vi "WinHostToFlexRIO.vi"() -> ()   [LabVIEW 2013]
uses:
  <vilib>/userdefined/High Color/nirio_resource_hc.ctl
  <vilib>/FPGAPlugInAG/PXIe-7966R/niLvFpga_Open_PXIe-7966R.vi
  <vilib>/FPGAPlugInAG/PXIe-7966R/niLvFpga_Reset_PXIe-7966R.vi
  <vilib>/FPGAPlugInAG/PXIe-7966R/niLvFpga_Run_PXIe-7966R.vi
  <vilib>/Utility/error.llb/Error Cluster From Error Code.vi
  <vilib>/rvi/errors/niLvFpgaAdjustHostInterfaceError.vi
  <vilib>/rvi/interface/common/niFpgaWaitOnOcc.vi
  <vilib>/FPGAPlugInAG/PXIe-7966R/niLvFpga_Close_PXIe-7966R.vi
  <vilib>/rvi/interface/nirviOpenFPGA/nirviOpenFPGA.xnode
  FPGA Bitfiles/PXIe-7966R-FlexRIOMod5761_v1_1.lvbitx
  FlexRIO5761.vi
  <vilib>/rvi/interface/nirviMethod/nirviMethod.xnode
  <vilib>/rvi/interface/nirviReadWriteControl/nirviReadWriteControl.xnode
  Control 1.ctl
  <vilib>/rvi/interface/nirviCloseFPGA/nirviCloseFPGA.xnode
  <vilib>/rvi/errors/niLvFpgaMergeErrorWithErrorCode.vi
  NiFpgaLv.dll
  <vilib>/FPGAPlugInAG/PXIe-7966R/niLvFpga_ReadFifo_PXIe-7966R.vi
  <vilib>/Analysis/NI_AALPro.lvlib
  <vilib>/FPGAPlugInAG/PXIe-7966R/niLvFpga_ConfigureFifo_PXIe-7966R.vi
  <vilib>/FPGAPlugInAG/PXIe-7966R/niLvFpga_StartFifo_PXIe-7966R.vi
panel:
  in  "SGSignalType1":enum16{"DC", "Sine", "Square", "Triangle"}(ring)
  out "Power spectrum graph":dynamicdata(graph)
  in  "SGAmp1":u16
  in  "AO1":i32
  in  "SGPhase1":u32
  in  "SGFreq1":u32
  in  "SGUpdateRate1":u32
  in  "AOEnable1":bool
  in  "FlexRIO device":T1
  out "DMA0 output":dynamicdata(graph)
  in  "SGSignalType0":enum16{"DC", "Sine", "Square", "Triangle"}(ring)
  in  "stop":bool
  out "auxAI9":i16
  out "SGNo":u8
  in  "SGAmp0":u16
  in  "SamplingRate0":u32=10000
  in  "DMATtoHOSTEnable0":bool
  in  "AO0":i16
  in  "SGFreq0":u32
  in  "SGPhase0":u32
  in  "SGUpdateRate0":u32=10000000
  in  "AOEnable0":bool
  in  "DebugMode":bool
  in  "DAQStartStop":bool
  out "error out":errorcluster
  out "DMATtoHOSTBlockNWords":u16[](array[numeric])
  out "DMATtoHOSTSampleSize":u8[](array[numeric])
  out "DMATtoHOSTNCh":u16[](array[numeric])
  out "DMATtoHOSTFrameType":u8[](array[numeric])
  out "DevProfile":u8
  out "DevTemp":i16
  out "DevQualityStatus":u8
  out "Fref":u32
  out "RIOAdapterCorrect":bool
  out "Expected IO Module ID":u32
  out "InsertedIOModule ID":u32
  out "FPGAVIversion":u8[](array[numeric])
  out "Platform":enum8{"FlexRIO", "cRIO", "RSeries"}(ring)
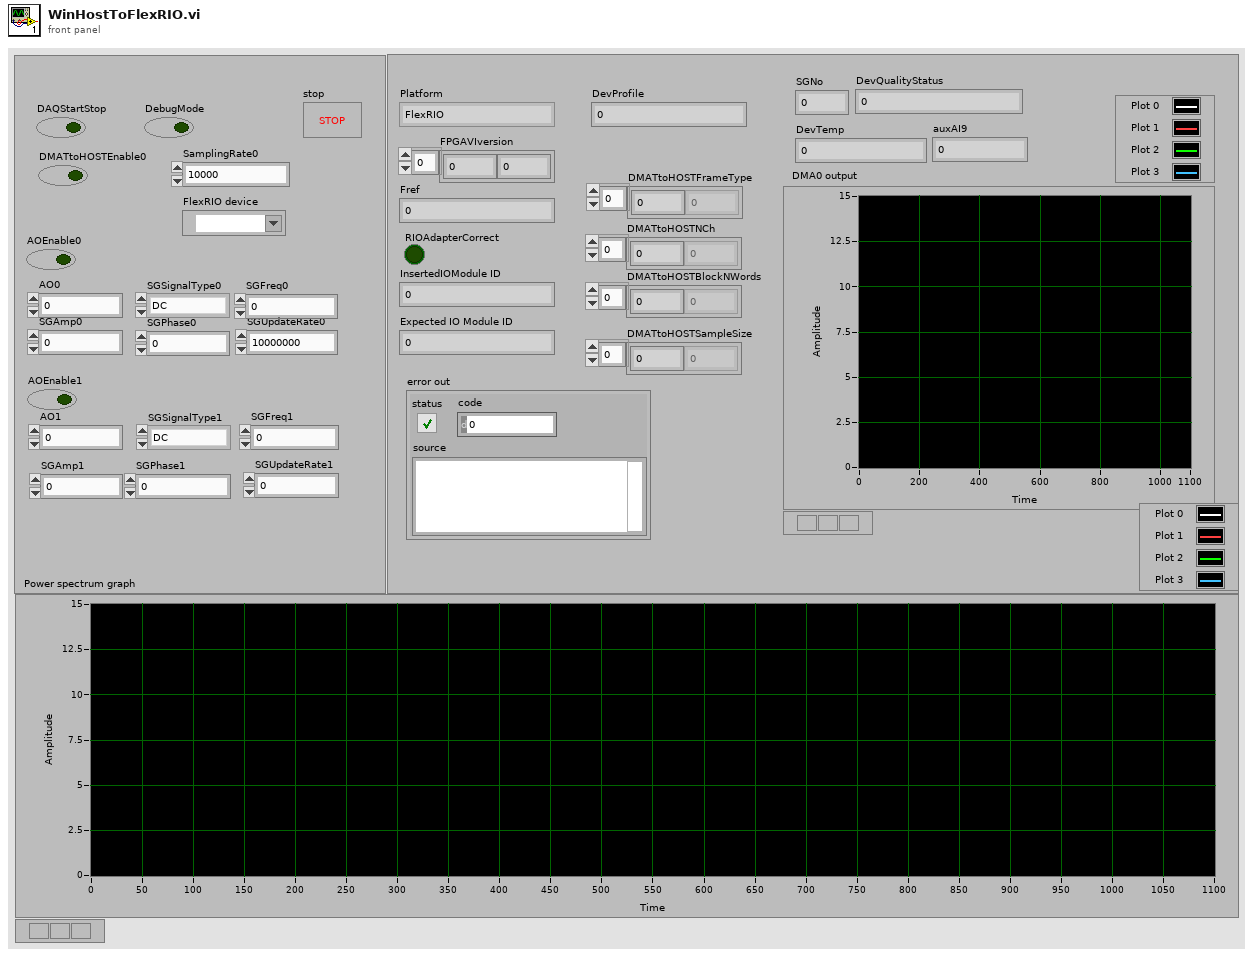
[diagram p1: front panel]
types:
  T1 = typedef "nirio_resource_hc.ctl" = tag
  T2 = enum16{"DAQ-CPU", "IMAQ-CPU", "DAQ-GPU", "IMAQ-GPU"}
  T3 = typedef "Control 1.ctl" = u16
  T4 = cluster{"Timeout":u8, "Timeout":T3, "Timeout":u8, "Timeout":u16}
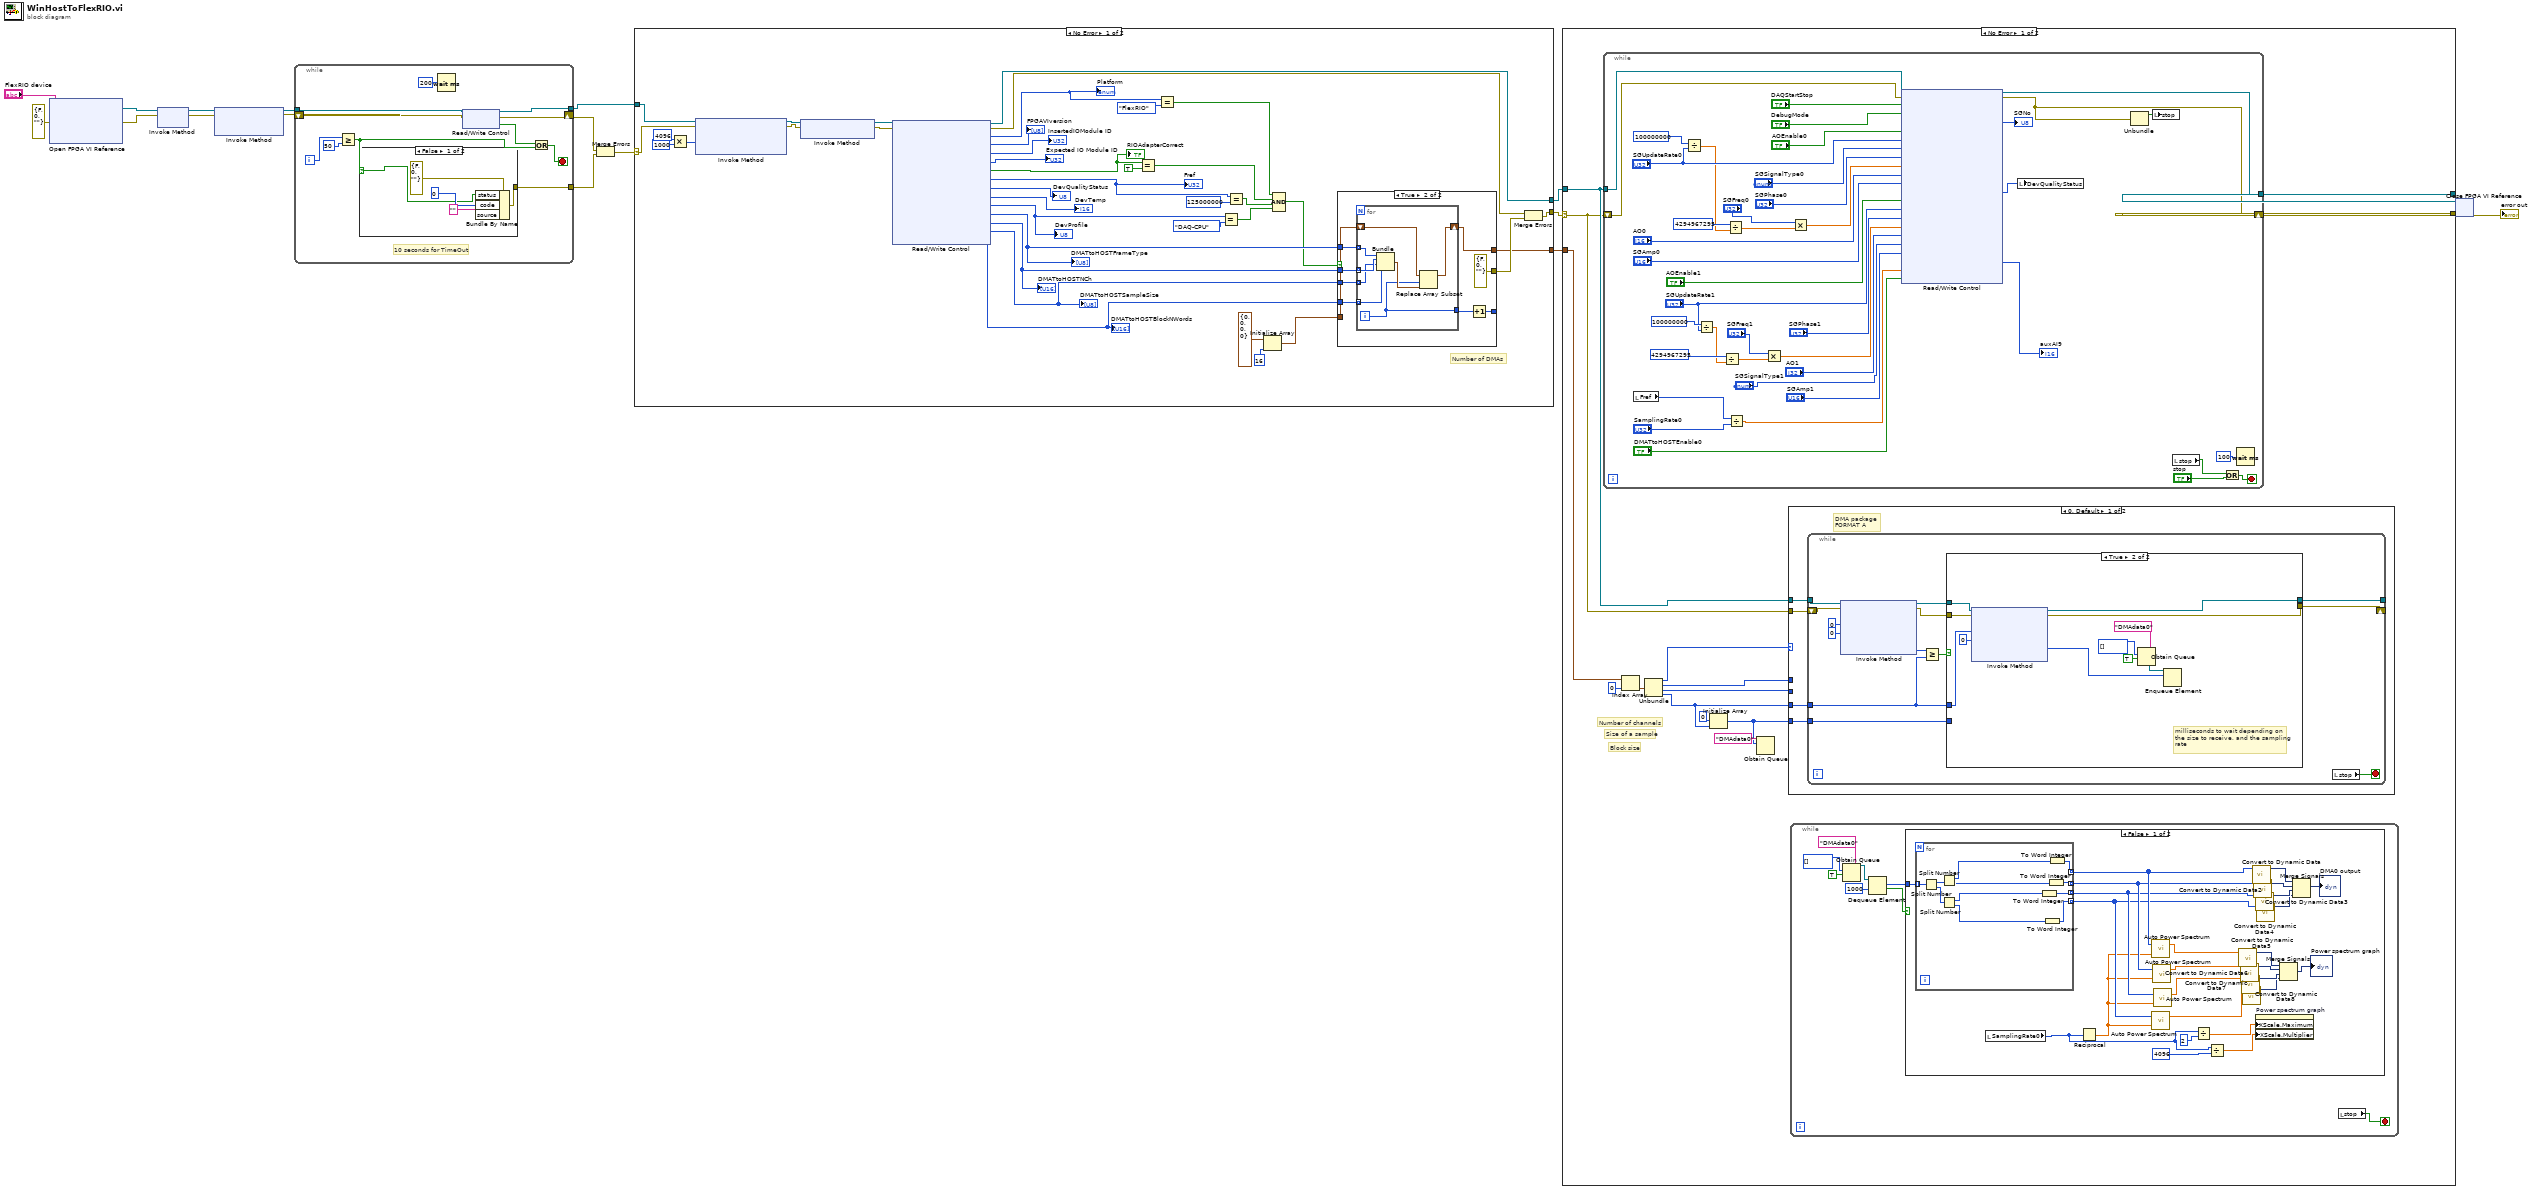
[diagram p0: block diagram]
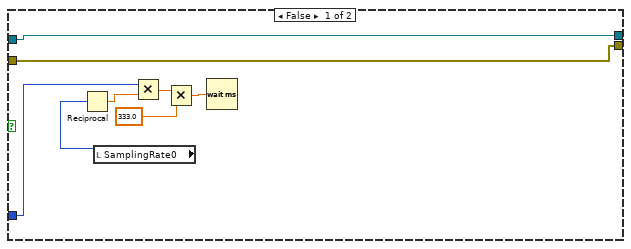
[diagram p3: hidden frame]
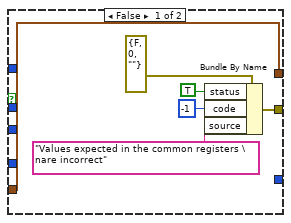
[diagram p6: hidden frame]
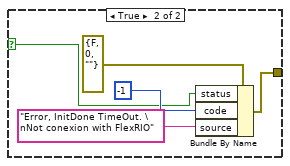
[diagram p8: hidden frame]
diagram:
  n1 = xnode "Open FPGA VI Reference"("error in"=errorcluster {"status"=FALSE, "code"=0, "source"=""}, "resource name"="FlexRIO device") -> ("FPGA VI Reference Out"=w15:refnum<k20>, "error out"=w16:errorcluster)
  n2 = xnode "Invoke Method"("FPGA VI Reference In"=w15, "error in"=w16) -> ("FPGA VI Reference Out"=w18:refnum<k20>, "error out"=w17:errorcluster)
  n3 = xnode "Invoke Method"("FPGA VI Reference In"=w18, "error in"=w17) -> ("FPGA VI Reference Out"=w13:refnum<k20>, "error out"=w12:errorcluster)  [unwired: 1 in]
  n4 = while {
    tunnel: w13 -> [w29]
    tunnel: [w26] -> w11
    shift-right: [w27] -> w9
    shift-left: w12 -> [w28]
    tunnel: [w19] -> w10
    i -> [w24]
    stop <- w21 stop-if-true
    # "10 seconds for TimeOut"
    n5 = Greater Or Equal?(x=w24, y=50) -> (x >= y?=w20:bool)
    n6 = case shown="False" w20 {
      selector: w20 -> [w31 w36]
      tunnel: [w30 w35] -> w19
      frame False {
        n7 = Bundle By Name(cluster=errorcluster {"status"=FALSE, "code"=0, "source"=""} ("error constant"), "status"=w31, "code"=0, "source"="") -> (w30:errorcluster)
      }
      frame True {
        n8 = Bundle By Name(cluster=errorcluster {"status"=FALSE, "code"=0, "source"=""} ("error constant"), "status"=w36, "code"=-1, "source"="Error, InitDone TimeOut. \nNot conexion with FlexRIO") -> (w35:errorcluster)
      }
    }
    n9 = Wait (ms)(milliseconds to wait=u32 200) -> ()  [unwired: 1 out]
    n10 = xnode "Read/Write Control"("FPGA VI Reference In"=w29, "error in"=w28) -> ("FPGA VI Reference Out"=w26:refnum<k20>, "error out"=w27:errorcluster, "InitDone"=w22:bool)
    n11 = Or(x=w22, y=w20) -> (x .or. y?=w21:bool)
  }
  n12 = Merge Errors(w9, w10) -> (w8:errorcluster)
  n13 = case shown="No Error" w8 {
    selector: w8 -> [w72 w103]
    tunnel: w11 -> [w73 w102]
    tunnel: [w67 w102] -> w5
    tunnel: [w43 w103] -> w6
    tunnel: [w41 _] -> w2
    frame No Error {
      # "Number of DMAs"
      n14 = Multiply(x=u32 4096 ("Requested Depth"), y=u32 1000) -> (x*y=w74:u32)
      n15 = xnode "Invoke Method"("FPGA VI Reference In"=w73, "error in"=w72, "Requested Depth"=w74) -> ("FPGA VI Reference Out"=w78:refnum<k20>, "error out"=w77:errorcluster)  [unwired: 1 out]
      n16 = xnode "Invoke Method"("FPGA VI Reference In"=w78, "error in"=w77) -> ("FPGA VI Reference Out"=w70:refnum<k20>, "error out"=w71:errorcluster)
      n17 = xnode "Read/Write Control"("FPGA VI Reference In"=w70, "error in"=w71) -> ("FPGA VI Reference Out"=w67:refnum<k20>, "error out"=w44:errorcluster, "Platform"=w66:enum8{"FlexRIO", "cRIO", "RSeries"}, "FPGAVIversion"=→"FPGAVIversion":u8[], "InsertedIOModule ID"=→"InsertedIOModule ID":u32, "Expected IO Module ID"=→"Expected IO Module ID":u32, "RIOAdapterCorrect"=w61:bool, "Fref"=w63:u32, "DevQualityStatus"=→"DevQualityStatus":u8, "DevTemp"=→"DevTemp":i16, "DevProfile"=w57:u8, "DMATtoHOSTFrameType"=w52:u8[], "DMATtoHOSTNCh"=w55:T3[], "DMATtoHOSTSampleSize"=w54:u8[], "DMATtoHOSTBlockNWords"=w53:u16[])
      "Platform" <- w66
      "RIOAdapterCorrect" <- w61
      "Fref" <- w63
      "DevProfile" <- w57
      "DMATtoHOSTFrameType" <- w52
      "DMATtoHOSTNCh" <- w55
      "DMATtoHOSTSampleSize" <- w54
      "DMATtoHOSTBlockNWords" <- w53
      n18 = Equal?(x=w61, y=TRUE) -> (x = y?=w50:bool)
      n19 = Equal?(x=w66, y=enum16{"FlexRIO", "cRIO", "R-Series"}."FlexRIO") -> (x = y?=w40:bool)
      n20 = Equal?(x=w57, y=T2."DAQ-CPU") -> (x = y?=w48:bool)
      n21 = Equal?(x=w63, y=u32 125000000) -> (x = y?=w49:bool)
      n22 = Initialize Array(cluster{u8, u16, u8, u16} {0, 0, 0, 0}, 16 ("dimension size")) -> (w45:cluster{u8, u16, u8, u16}[])
      n23 = Compound Arithmetic op=AND(w40, w50, w49, w48) -> (w51:bool)
      n24 = case shown="True" w51 {
        tunnel: w55 -> [_ w93]
        tunnel: w54 -> [_ w92]
        tunnel: w53 -> [_ w91]
        tunnel: w52 -> [_ w90]
        tunnel: w45 -> [w79 w89]
        tunnel: [w79 w88] -> w41
        tunnel: [w80 errorcluster {"status"=FALSE, "code"=0, "source"=""} ("error constant")] -> w42
        tunnel: [_ w85] -> _
        frame False {
          n25 = Bundle By Name(cluster=errorcluster {"status"=FALSE, "code"=0, "source"=""} ("error constant"), "status"=TRUE, "code"=-1, "source"="Values expected in the common registers \nare incorrect") -> (w80:errorcluster)
        }
        frame True {
          n26 = for {
            tunnel: w93 -> [w99] mode=indexing
            tunnel: w92 -> [w98] mode=indexing
            tunnel: w91 -> [w97] mode=indexing
            tunnel: w90 -> [w100] mode=indexing
            shift-right: [w95] -> w88
            shift-left: w89 -> [w101]
            tunnel: [w94] -> w86
            i -> [w94]
            n27 = Bundle("Timeout"=w100, "Timeout"=w99, "Timeout"=w98, "Timeout"=w97) -> (w96:T4)  [unwired: 1 in]
            n28 = Replace Array Subset(array=w101, new element=w96, index=w94) -> (w95:cluster{u8, u16, u8, u16}[])
          }
          n29 = Increment(x=w86) -> (x+1=w85:i32)
        }
      }
      n30 = Merge Errors(w44, w42) -> (w43:errorcluster)
    }
    frame Error {
    }
  }
  n31 = case shown="No Error" w6 {
    selector: w6 -> [w109 w241]
    tunnel: w5 -> [w110 w240]
    tunnel: [w117 w240] -> w4
    tunnel: [w116 w241] -> w3
    tunnel: w2 -> [w115 _]
    frame No Error {
      # "Block size"
      # "Size of a sample"
      # "Number of channels"
      n32 = while {
        shift-right: [w226] -> w116
        shift-left: w109 -> [w238]
        tunnel: w110 -> [w239]
        tunnel: [w237] -> w117
        stop <- w228 stop-if-true
        n33 = local read "Fref"() -> (w221:u32)
        n34 = Divide(x=100000000, y="SGUpdateRate0") -> (x/y=w212:dbl)
        n35 = Divide(x=100000000, y="SGUpdateRate1") -> (x/y=w204:dbl)
        n36 = Divide(x=i64 4294967295, y=w204) -> (x/y=w206:dbl)
        n37 = Divide(x=i64 4294967295, y=w212) -> (x/y=w216:dbl)
        n38 = Divide(x=w221, y="SamplingRate0") -> (x/y=w222:dbl)
        n39 = Multiply(x="SGFreq1", y=w206) -> (x*y=w202:dbl)
        n40 = Multiply(x="SGFreq0", y=w216) -> (x*y=w214:dbl)
        n41 = xnode "Read/Write Control"("FPGA VI Reference In"=w239, "error in"=w238, "DAQStartStop"="DAQStartStop", "DebugMode"="DebugMode", "AOEnable0"="AOEnable0", "SGUpdateRate0"="SGUpdateRate0", "SGSignalType0"="SGSignalType0", "SGPhase0"="SGPhase0", "SGFreq0"=w214, "AO0"="AO0", "SGAmp0"="SGAmp0", "AOEnable1"="AOEnable1", "SGUpdateRate1"="SGUpdateRate1", "SGPhase1"="SGPhase1", "SGFreq1"=w202, "AO1"="AO1", "SGSignalType1"="SGSignalType1", "SGAmp1"="SGAmp1", "DMATtoHOSTSamplingRate0"=w222, "DMATtoHOSTEnable0"="DMATtoHOSTEnable0") -> ("FPGA VI Reference Out"=w237:refnum<k20>, "error out"=w226:errorcluster, "SGNo"=→"SGNo":u8, "DevQualityStatus"=w230:u8, "auxAI9"=→"auxAI9":i32)
        n42 = local write "DevQualityStatus"(w230) -> ()
        n43 = Unbundle(w226) -> ("status"=w225:bool)  [unwired: 2 out]
        n44 = local write "stop"(w225) -> ()
        n45 = local read "stop"() -> (w224:bool)
        n46 = Or(x=w224, y="stop") -> (x .or. y?=w228:bool)
        n47 = Wait (ms)(milliseconds to wait=u32 100) -> ()  [unwired: 1 out]
      }
      n48 = Index Array(array=w115, index=0) -> (element=w113:cluster{u8, u16, u8, u16})
      n49 = Unbundle(w113) -> (w112:u8, w111:u16, w108:u8, w106:u16)
      n50 = Initialize Array(u64 0, w106) -> (w104:u64[])
      n51 = Obtain Queue(name (unnamed)="DMAdata0", element data type=w104) -> ()  [unwired: 3 in, 3 out]
      n52 = case shown="0, Default" w112 {
        tunnel: w111 -> [_ _]
        tunnel: w108 -> [_ _]
        tunnel: w106 -> [w162 _]
        tunnel: w110 -> [w165 _]
        tunnel: w109 -> [w163 _]
        tunnel: w104 -> [w164 _]
        frame 0, Default {
          # "DMA package \nFORMAT A"
          n53 = while {
            tunnel: w165 -> [w175]
            tunnel: w164 -> [w168]
            tunnel: w162 -> [w170]
            tunnel: [w177] -> _
            shift-right: [w176] -> _
            shift-left: w163 -> [w174]
            stop <- w178 stop-if-true
            n54 = xnode "Invoke Method"("FPGA VI Reference In"=w175, "error in"=w174, "Number of Elements"=u32 0, "Timeout (ms)"=0) -> ("FPGA VI Reference Out"=w167:refnum<k20>, "error out"=w166:errorcluster, "Elements Remaining"=w171:u32)  [unwired: 1 out]
            n55 = Greater Or Equal?(x=w171, y=w170) -> (x >= y?=w169:bool)
            n56 = case shown="True" w169 {
              tunnel: [w180 w197] -> w177
              tunnel: [w179 w196] -> w176
              tunnel: w170 -> [w182 w195]
              tunnel: w168 -> [_ _]
              tunnel: w167 -> [w180 w188]
              tunnel: w166 -> [w179 w187]
              frame False {
                n57 = local read "SamplingRate0"() -> (w181:u32)
                n58 = Reciprocal(x=w181) -> (1/x=w186:dbl)
                n59 = Multiply(x=w182, y=w186) -> (x*y=w185:dbl)
                n60 = Multiply(x=w185, y=333.0) -> (x*y=w183:dbl)
                n61 = Wait (ms)(milliseconds to wait=w183) -> ()  [unwired: 1 out]
              }
              frame True {
                # "milliseconds to wait depending on \nthe size to receive, and the sampling\nrate"
                n62 = xnode "Invoke Method"("FPGA VI Reference In"=w188, "error in"=w187, "Number of Elements"=w195, "Timeout (ms)"=0) -> ("FPGA VI Reference Out"=w197:refnum<k20>, "error out"=w196:errorcluster, "Data"=w189:u64[])  [unwired: 1 out]
                n63 = Obtain Queue(name (unnamed)="DMAdata0", element data type=u64[] [], create if not found? (T)=TRUE) -> (queue out=w193:refnum<queue>)  [unwired: 2 in, 2 out]
                n64 = Enqueue Element(queue=w193, element=w189) -> ()  [unwired: 2 in, 3 out]
              }
            }
            n65 = local read "stop"() -> (w178:bool)
          }
        }
        frame 1 {
        }
      }
      n66 = while {
        stop <- w120 stop-if-true
        n67 = Obtain Queue(name (unnamed)="DMAdata0", element data type=u64[] [], create if not found? (T)=TRUE) -> (queue out=w122:refnum<queue>)  [unwired: 2 in, 2 out]
        n68 = Dequeue Element(queue=w122, timeout in ms (-1)=1000) -> (element=w121:u64[], timed out?=w118:bool)  [unwired: 1 in, 2 out]
        n69 = case shown="False" w118 {
          tunnel: w121 -> [w150 _]
          frame False {
            n70 = for {
              tunnel: w150 -> [w161] mode=indexing
              tunnel: [w151] -> w139 mode=indexing
              tunnel: [w153] -> w137 mode=indexing
              tunnel: [w155] -> w134 mode=indexing
              tunnel: [w157] -> w133 mode=indexing
              n71 = Split Number(x=w161) -> (hi(x)=w160:u32, lo(x)=w159:u32)
              n72 = Split Number(x=w160) -> (hi(x)=w152:u16, lo(x)=w154:u16)
              n73 = Split Number(x=w159) -> (hi(x)=w156:u16, lo(x)=w158:u16)
              n74 = To Word Integer(number=w156) -> (16bit integer=w155:i16)
              n75 = To Word Integer(number=w158) -> (16bit integer=w157:i16)
              n76 = To Word Integer(number=w154) -> (16bit integer=w153:i16)
              n77 = To Word Integer(number=w152) -> (16bit integer=w151:i16)
            }
            n78 = local read "SamplingRate0"() -> (w129:u32)
            n79 = Reciprocal(x=w129) -> (1/x=w131:dbl)
            n80 = call <vilib>:"Auto Power Spectrum.vi"("dt"=w131, "Signal (V)"=w139) -> ("Power Spectrum (V^2 rms)"=w138:dbl[])  [unwired: 1 out]
            n81 = call <vilib>:"Auto Power Spectrum.vi"("dt"=w131, "Signal (V)"=w133) -> ("Power Spectrum (V^2 rms)"=w132:dbl[])  [unwired: 1 out]
            n82 = call <vilib>:"Auto Power Spectrum.vi"("dt"=w131, "Signal (V)"=w137) -> ("Power Spectrum (V^2 rms)"=w136:dbl[])  [unwired: 1 out]
            n83 = call <vilib>:"Auto Power Spectrum.vi"("dt"=w131, "Signal (V)"=w134) -> ("Power Spectrum (V^2 rms)"=w135:dbl[])  [unwired: 1 out]
            n84 = Divide(x=w129, y=2) -> (x/y=w126:dbl)
            n85 = Divide(x=w129, y=4096) -> (x/y=w127:dbl)
            n86 = call "Convert to Dynamic Data5"("Array"=w138) -> ("Dynamic Data Type"=w144:dynamicdata)  [unwired: 3 in]
            n87 = call "Convert to Dynamic Data6"("Array"=w136) -> ("Dynamic Data Type"=w143:dynamicdata)  [unwired: 3 in]
            n88 = call "Convert to Dynamic Data7"("Array"=w135) -> ("Dynamic Data Type"=w142:dynamicdata)  [unwired: 3 in]
            n89 = call "Convert to Dynamic Data8"("Array"=w132) -> ("Dynamic Data Type"=w141:dynamicdata)  [unwired: 3 in]
            n90 = call "Convert to Dynamic Data"("Array"=w139) -> ("Dynamic Data Type"=w148:dynamicdata)  [unwired: 3 in]
            n91 = call "Convert to Dynamic Data2"("Array"=w137) -> ("Dynamic Data Type"=w147:dynamicdata)  [unwired: 3 in]
            n92 = call "Convert to Dynamic Data3"("Array"=w134) -> ("Dynamic Data Type"=w146:dynamicdata)  [unwired: 3 in]
            n93 = property on="Power spectrum graph" class="WFGraph (strict)"("XScale.Maximum"=w126, "XScale.Multiplier"=w127) -> ()  [unwired: 2 in, 2 out]
            n94 = call "Convert to Dynamic Data4"("Array"=w133) -> ("Dynamic Data Type"=w145:dynamicdata)  [unwired: 3 in]
            n95 = Merge Signals(w144, w143, w142, w141) -> (→"Power spectrum graph":dynamicdata)
            n96 = Merge Signals(w148, w147, w146, w145) -> (→"DMA0 output":dynamicdata)
          }
          frame True {
          }
        }
        n97 = local read "stop"() -> (w120:bool)
      }
    }
    frame Error {
    }
  }
  n98 = xnode "Close FPGA VI Reference"("FPGA VI Reference In"=w4, "error in"=w3) -> ("error out"=→"error out":errorcluster)
